vi "From Listener.vi"(7 "From":refnum<class "Endpoint.lvclass">, 8 "error in (no error)":errorcluster, 9 "TCP Connection":refnum<k5>, 10 "URI":refnum<class "URI.lvclass">, 11 "Client Type":refnum<class "TCP Client.lvclass">) -> (0 "error out":errorcluster, 3 "TCP Client":refnum<class "TCP Client.lvclass">)   [LabVIEW 2020, in "Stream-TCP.lvlib" / "TCP Client.lvclass"]
uses:
  TCP Client.lvclass
  <vilib>/IlluminatedG/lv-stream/URI/URI.lvclass
  C:/Program Files (x86)/National Instruments/LabVIEW 2020/vi.lib/IlluminatedG/lv-stream/Endpoint/Endpoint.lvclass
  C:/Program Files (x86)/National Instruments/LabVIEW 2020/vi.lib/IlluminatedG/lv-stream/Connection/Connection.lvclass
  <vilib>/IlluminatedG/lv-stream/Endpoint/Endpoint.lvclass
  <vilib>/IlluminatedG/lv-stream/Connection State.ctl
  <vilib>/IlluminatedG/lv-stream/Connection/State.ctl
  <vilib>/IlluminatedG/lv-stream/Stream.lvlib
  <vilib>/IlluminatedG/lv-stream/Connection/Connection.lvclass
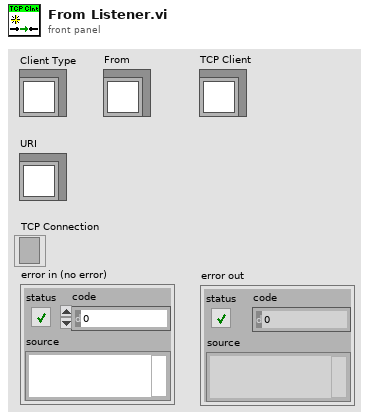
[diagram p1: front panel]
types:
  T1 = typedef "Stream.lvlib/Connection.lvclass/State.ctl" = enum16{"Closed", "Idle", "Connecting", "Connected", "Shutdown"}
  T2 = typedef "Stream.lvlib/Connection State.ctl" = enum16{"Connected", "Disconnected"}
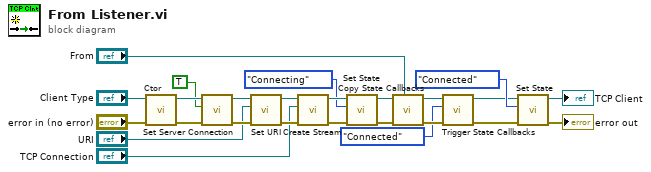
[diagram p0: block diagram]
diagram:
  n1 = call-dynamic "Ctor.vi"("error in (no error)"="error in (no error)", "TCP Client in"="Client Type") -> ("error out"=w18:errorcluster, "TCP Client out"=w19:refnum<class "TCP Client.lvclass">)  [unwired: 8 in]
  n2 = call "Set Server Connection.vi"("error in (no error)"=w18, "Is Server Connection"=TRUE ("Server Connection"), "TCP Client in"=w19) -> ("error out"=w25:errorcluster, "TCP Client out"=w2:refnum<class "TCP Client.lvclass">)  [unwired: 7 in]
  n3 = call <vilib>:"Set URI.vi"("error in (no error)"=w25, "URI"="URI", "Endpoint in"=w2) -> ("error out"=w24:errorcluster, "Endpoint out"=w8:refnum<class "TCP Client.lvclass">)  [unwired: 7 in]
  n4 = call "Create Stream.vi"("error in (no error)"=w24, "TCP Connection"="TCP Connection", "TCP Client in"=w8) -> ("error out"=w14:errorcluster, "TCP Client out"=w15:refnum<class "TCP Client.lvclass">)  [unwired: 7 in]
  n5 = call <vilib>:"Set State.vi"("error in (no error)"=w14, "State"=State."Connecting", "Connection in"=w15) -> ("error out"=w13:errorcluster, "Connection out"=w12:refnum<class "TCP Client.lvclass">)  [unwired: 7 in]
  n6 = call <vilib>:"Copy State Callbacks.vi"("From"="From", "error in (no error)"=w13, "Endpoint in"=w12) -> ("error out"=w22:errorcluster, "Endpoint out"=w23:refnum<class "TCP Client.lvclass">)  [unwired: 7 in]
  n7 = call <vilib>:"Trigger State Callbacks.vi"("error in (no error)"=w22, "State"=Connection_State."Connected", "Connection in"=w23) -> ("error out"=w5:errorcluster, "Connection out"=w6:refnum<class "TCP Client.lvclass">)  [unwired: 7 in]
  n8 = call <vilib>:"Set State.vi"("error in (no error)"=w5, "State"=State."Connected", "Connection in"=w6) -> ("error out"=→"error out":errorcluster, "Connection out"=→"TCP Client":refnum<class "TCP Client.lvclass">)  [unwired: 7 in]
